vi "FRC myRIO v1.0 Configure I2C.vi"(8 "error in (no error)":errorcluster, 9 "I2C Counter Value":u8) -> (0 "error out":errorcluster)   [LabVIEW 2017]
uses:
  <vilib>/rvi/errors/niLvFpgaAdjustHostInterfaceError.vi
  <vilib>/Utility/error.llb/Error Cluster From Error Code.vi
  <vilib>/Rock Robotics/SystemInterfaces/System/FPGA_SystemFRC FPGA Ref.ctl
  <vilib>/rvi/interface/nirviReadWriteControl/nirviReadWriteControl.xnode
  NiFpgaLv.dll
  <vilib>/rvi/interface/Simulation/niFpgaSimulationCallBeginRW.vi
panel:
  # "This VI configures the I2C counter register (I2C.n_0.CNTR) based on the value of the I2C Transfer Rate control and sets bit 0 of the configuration register (I2C.n_0.CNFG) to enable the I2C master logic in the FPGA.\nPlease see Block Diagram for details."
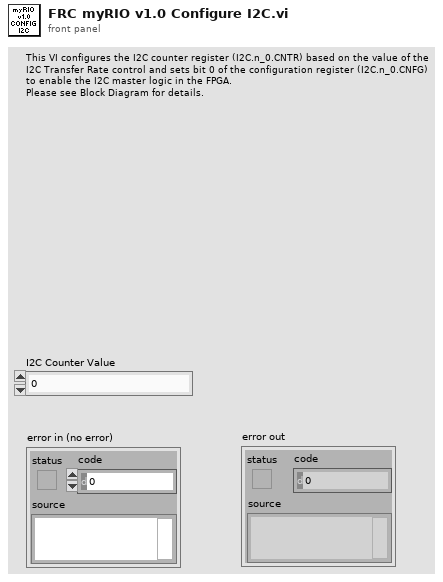
[diagram p1: front panel]
types:
  T1 = typedef "FPGA_SystemFRC FPGA Ref.ctl" = refnum<k20>
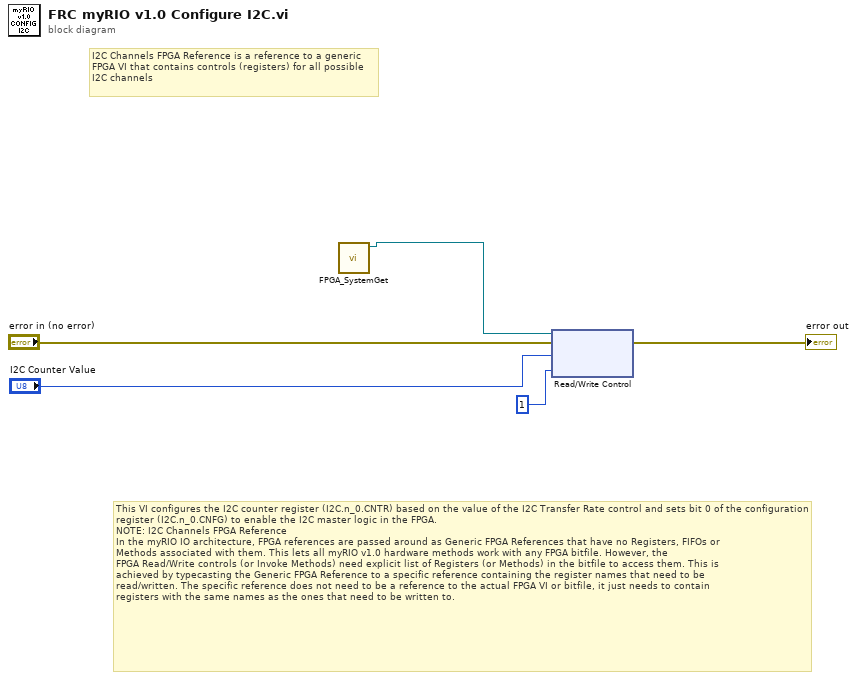
[diagram p0: block diagram]
diagram:
  # "This VI configures the I2C counter register (I2C.n_0.CNTR) based on the value of the I2C Transfer Rate control and sets bit 0 of the configuration register (I2C.n_0.CNFG) to enable the I2C master logic in the FPGA.\nNOTE: I2C Channels FPGA Reference\nIn the myRIO IO architecture, FPGA references are passed around as Generic FPGA References that have no Registers, FIFOs or\nMethods associated with them. This lets all myRIO v1.0 hardware methods work with any FPGA bitfile. However, the \nFPGA Read/Write controls (or Invoke Methods) need explicit list of Registers (or Methods) in the bitfile to access them. This is \nachieved by typecasting the Generic FPGA Reference to a specific reference containing the register names that need to be \nread/written. The specific reference does not need to be a reference to the actual FPGA VI or bitfile, it just needs to contain \nregisters with the same names as the ones that need to be written to."
  # "I2C Channels FPGA Reference is a reference to a generic FPGA VI that contains controls (registers) for all possible I2C channels"
  n1 = call <vilib>:"FPGA_SystemGet.vi"() -> ("FRC FPGA Ref"=w2:T1)  [unwired: 11 in]
  n2 = xnode "Read/Write Control"("FPGA VI Reference In"=w2, "error in"="error in (no error)", "Accel.CNTR"="I2C Counter Value", "Accel.CNFG"=u8 1 ("I2C0.CNFG")) -> ("error out"=→"error out":errorcluster)  [unwired: 1 out]
